vi "6.4.-Lógica Difusa con Arrays Carrito - Giro y Seguimiento de Mouse.vi"() -> ()   [LabVIEW 2020]
uses:
  <vilib>/addons/Fuzzy Logic/FL Fuzzy Controller (MIMO).vi
  <vilib>/addons/Fuzzy Logic/NI_Fuzzy_Logic_API.lvlib
panel:
  out "Motor derecho":dbl[][](array[numeric])
  out "Motor Izquerdo":dbl[][](array[numeric])
  out "Distancia":dbl(slide) scale=0.0..100.0
  out "Angulo":dbl(knob) scale=-25.0..25.0
  in  "Reset":bool
  out "Motor Izquierda":dbl(slide) scale=-100.0..100.0
  out "Motor Derecha":dbl(slide) scale=-100.0..100.0
  out "Plano de trabajo":picture
  in  "stop":bool
  # "En este VI ya no solamente apuntará el carrito a donde estará el mouse sino que lo seguirá"
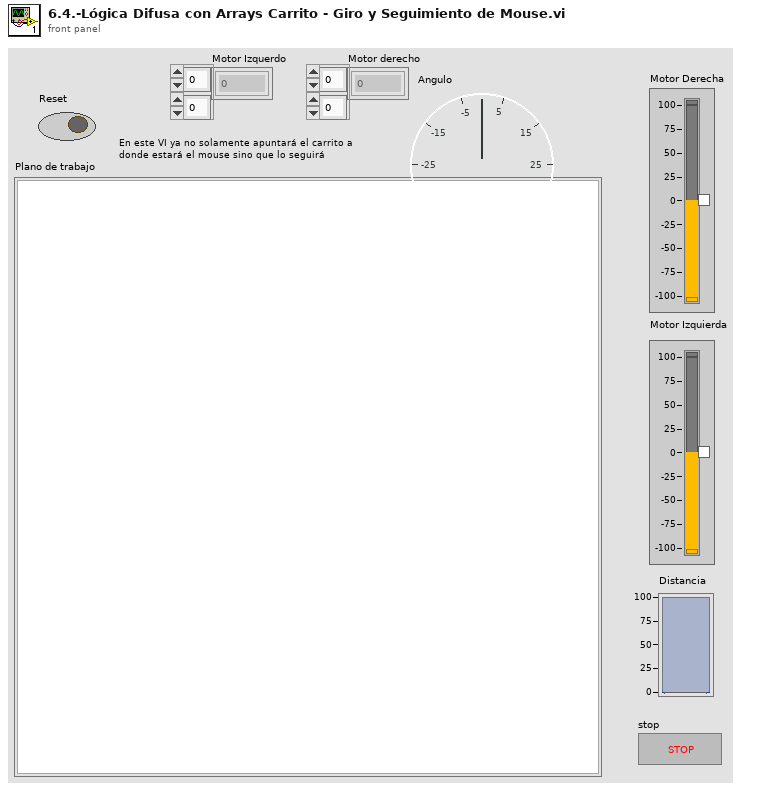
[diagram p1: front panel]
types:
  T1 = typedef "NI_Fuzzy_Logic_API.lvlib/FL System.ctl" = cluster{"input variables":T2[], "output variables":T2[], "rules":T5[], "defuzzification method":T11, "description":string, "user MF interpolating polynomials":T12[]}
  T2 = typedef "NI_Fuzzy_Logic_API.lvlib/FL Variable.ctl" = cluster{"name":string, "range":dbl[], "MFs":T3[]}
  T3 = typedef "NI_Fuzzy_Logic_API.lvlib/FL Membership Function.ctl" = cluster{"name":string, "shape":T4, "points":dbl[], "color":u32, "user-defined shape index":i32}
  T4 = typedef "NI_Fuzzy_Logic_API.lvlib/FL Membership Function Shape.ctl" = u16
  T5 = typedef "NI_Fuzzy_Logic_API.lvlib/FL Rule.ctl" = cluster{"antecedents":T6[], "antecedent connective":T8, "consequents":T9[], "consequent implication":T10, "degree of support":dbl}
  T6 = typedef "NI_Fuzzy_Logic_API.lvlib/FL Antecedent.ctl" = cluster{"Var Index":i32, "MF Index":i32, "Cond":T7}
  T7 = typedef "NI_Fuzzy_Logic_API.lvlib/FL Modifier.ctl" = u16
  T8 = typedef "NI_Fuzzy_Logic_API.lvlib/FL Antecedent Connective.ctl" = u16
  T9 = typedef "NI_Fuzzy_Logic_API.lvlib/FL Consequent.ctl" = cluster{"Var Index":i32, "MF Index":i32, "Cond":T7}
  T10 = typedef "NI_Fuzzy_Logic_API.lvlib/FL Consequent Implication.ctl" = u16
  T11 = typedef "NI_Fuzzy_Logic_API.lvlib/FL Defuzzification.ctl" = u16
  T12 = typedef "NI_Fuzzy_Logic_API.lvlib/FL Interpolating polynomials.ctl" = cluster{"X":dbl[], "Y":dbl[], "Y(x) coeff":dbl[][], "X(y) coeff":dbl[][], "Area(y) coeff":dbl[][], "coa_x(y) coeff":dbl[][]}
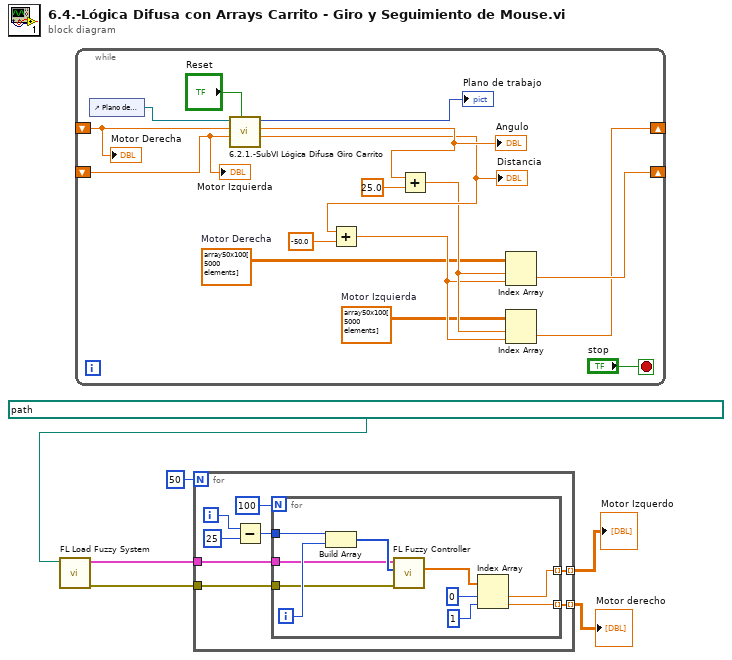
[diagram p0: block diagram]
diagram:
  n1 = call <vilib>:"FL Load Fuzzy System.vi"("file path"=path "C:/Users/diego/OneDrive/Documents/Aprendiendo/LabVIEW/1.-Sistemas de Visión Artificial/6.3.0.-Modelo Lógica Difusa Giro y Seguimiento Carrito.fs") -> ("error out"=w4:errorcluster, "fuzzy system out"=w3:T1)  [unwired: 9 in]
  n2 = while {
    shift-right: [w18] -> _
    shift-left: _ -> [w15]
    shift-right: [w17] -> _
    shift-left: _ -> [w16]
    stop <- "stop" stop-if-true
    w7 = dbl[][] array50x100[5000 elements]  # Motor Izquierda
    w8 = dbl[][] array50x100[5000 elements]  # Motor Derecha
    n3 = control-ref of="Plano de trabajo"() -> (w20:refnum<vi>)
    n4 = call "6.2.1.-SubVI Lógica Difusa Giro Carrito.vi"("Reset"="Reset", "Motor Izquierda"=w15, "Motor Derecha"=w16, "Ref Plano"=w20) -> ("Distancia"=w11:dbl, "Angulo"=w13:dbl, "Plano de trabajo"=→"Plano de trabajo":picture)  [unwired: 3 in, 2 out]
    "Angulo" <- w13
    "Distancia" <- w11
    n5 = Add(x=w11, y=-50.0) -> (x+y=w9:dbl)
    n6 = Add(x=w13, y=25.0) -> (x+y=w10:dbl)
    n7 = Index Array "Index Array"(array=w8, index (row)=w10, index (col)=w9) -> (element=w18:dbl)
    n8 = Index Array "Index Array"(array=w7, index (row)=w10, index (col)=w9) -> (element=w17:dbl)
    "Motor Derecha" <- w16
    "Motor Izquierda" <- w15
  }
  n9 = for {
    N: 50 -> [_]
    tunnel: [w30] -> w1 mode=indexing
    tunnel: [w29] -> w6 mode=indexing
    tunnel: w4 -> [w25]
    tunnel: w3 -> [w24]
    i -> [w26]
    n10 = Subtract(x=w26, y=25) -> (x-y=w23:i32)
    n11 = for {
      N: 100 -> [_]
      tunnel: [w37] -> w30 mode=indexing
      tunnel: [w36] -> w29 mode=indexing
      tunnel: w25 -> [w33]
      tunnel: w24 -> [w32]
      tunnel: w23 -> [w31]
      i -> [w35]
      n12 = Build Array "Build Array"(w31, w35) -> (w34:i32[])
      n13 = call-poly <vilib>:"FL Fuzzy Controller.vi"("error in (no error)"=w33, "input values"=w34, "fuzzy system in"=w32) -> ("output values"=w40:dbl[])  [unwired: 4 in, 4 out]
      n14 = Index Array "Index Array"(array=w40, index #1=0 ("index"), index #2=1 ("index")) -> (element #1=w37:dbl, element #2=w36:dbl)
    }
  }
  "Motor Izquerdo" <- w1
  "Motor derecho" <- w6
